vi "FdxCmdTxUDPDestroyPortCvi.vi"(8 "error in":errorcluster, 10 "UdpHandle":u32, 11 "InstrumentHandle":u32) -> (0 "error out":errorcluster, 3 "InstrumentHandle":u32)   [LabVIEW 2020, in "AIM664LV.lvlib"]
doc: "This function is used to destroy the UDP transmit port, if it is no longer in use. (This function is the opposite of function to AiFdxCmdTxUDPCreatePort and AiFdxCmdTxSAPCreatePort.) This function can be used only when transmitter is not running."
uses:
  AIM664LV.lvlib
  AFDX_LibraryAdmin/FdxGlobalDllPath.vi
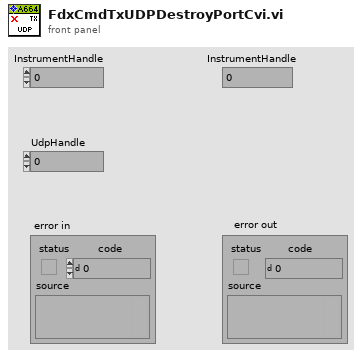
[diagram p1: front panel]
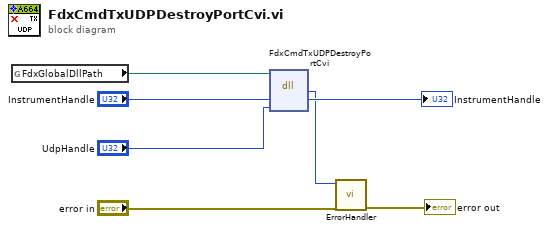
[diagram p0: block diagram]
diagram:
  n1 = global read "FdxGlobalDllPath.vi" "FdxGlobalDllPath"() -> (w5:path)
  n2 = dll-call lib="aim_fdx.19.dll" fn="FdxCmdTxUDPDestroyPortCvi"(path in=w5, "InstrumentHandle"="InstrumentHandle", "UdpHandle"="UdpHandle") -> ("status"=w1:i32, "InstrumentHandle"=→"InstrumentHandle":u32)  [unwired: 3 in, 2 out]
  n3 = call "ErrorHandler.vi"("error in"="error in", "AIM Error"=w1) -> ("error out"=→"error out":errorcluster)  [unwired: 9 in]
